vi "read parameters limits.vi"(8 "error in (no error)":errorcluster, 11 "Simulated_CCD_Camera in":refnum<class "Simulated_CCD_Camera.lvclass">) -> (0 "error out":errorcluster, 2 "limit values spreadsheet":string[][](array[string]), 3 "Simulated_CCD_Camera out":refnum<class "Simulated_CCD_Camera.lvclass">)   [LabVIEW 2018, in "Simulated_CCD_Camera.lvclass"]
uses:
  Simulated_CCD_Camera.lvclass
  <vilib>/Utility/file.llb/Read Delimited Spreadsheet (string).vi
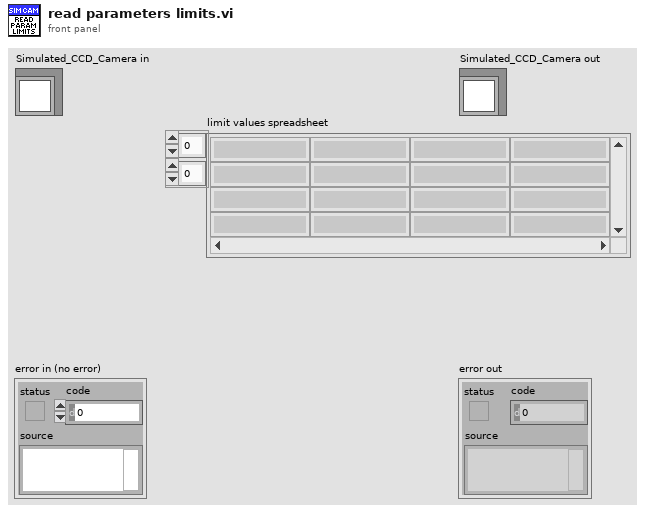
[diagram p1: front panel]
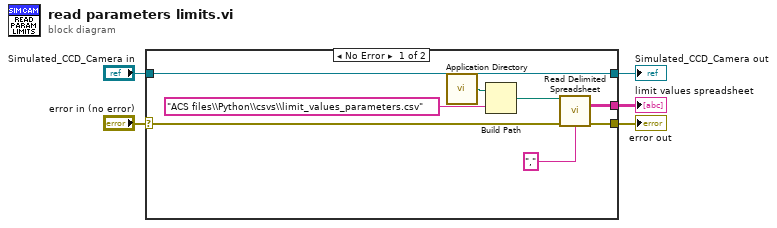
[diagram p0: block diagram]
diagram:
  n1 = case shown="No Error" "error in (no error)" {
    selector: "error in (no error)" -> [w8 w15]
    tunnel: [w7 w15] -> w4
    tunnel: [w13 w14] -> w2
    tunnel: "Simulated_CCD_Camera in" -> [w13 w14]
    tunnel: [w6 _] -> w1
    frame No Error {
      n2 = call <vilib>:"Application Directory.vi"() -> ("Application Directory"=w10:path)
      n3 = Build Path(base path=w10, name or relative path="ACS files\\Python\\csvs\\limit_values_parameters.csv") -> (appended path=w11:path)
      n4 = call-poly <vilib>:"Read Delimited Spreadsheet.vi"("file path (dialog if empty)"=w11, "error in (no error)"=w8, "delimiter (\\t)"="," ("delimiter (\\t)")) -> ("all rows"=w6:string[][], "error out"=w7:errorcluster)  [unwired: 7 in, 4 out]
    }
    frame Error {
    }
  }
  "error out" <- w4
  "Simulated_CCD_Camera out" <- w2
  "limit values spreadsheet" <- w1
